vi "Straight Drive.vi"(0 "X":dbl, 1 "Y":dbl, 2 "Z":dbl, 3 "Straight?":bool, 4 "Reverse?":bool) -> (5 "Axes Magnitudes":cluster{"X":dbl, "Y":dbl, "Z":dbl})   [LabVIEW 2016]
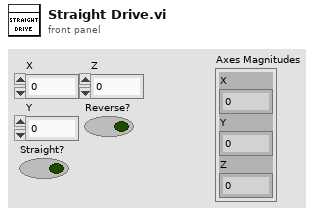
[diagram p1: front panel]
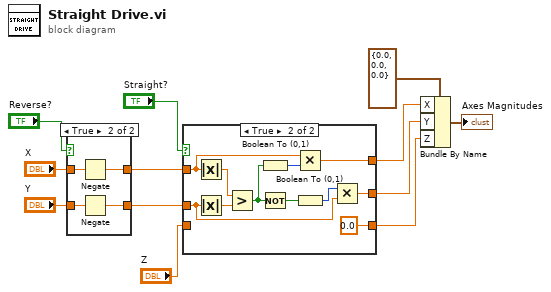
[diagram p0: block diagram]
diagram:
  n1 = case shown="True" "Reverse?" {
    tunnel: [w14 w16] -> w6
    tunnel: "X" -> [w14 w18]
    tunnel: [w13 w17] -> w7
    tunnel: "Y" -> [w13 w15]
    frame False {
    }
    frame True {
      n2 = Negate(x=w18) -> (-x=w16:dbl)
      n3 = Negate(x=w15) -> (-x=w17:dbl)
    }
  }
  n4 = case shown="True" "Straight?" {
    tunnel: w6 -> [w21 w30]
    tunnel: w7 -> [w20 w25]
    tunnel: "Z" -> [w19 _]
    tunnel: [w21 w32] -> w11
    tunnel: [w19 0.0] -> w8
    tunnel: [w20 w31] -> w10
    frame False {
    }
    frame True {
      n5 = Absolute Value(x=w30) -> (abs(x)=w24:dbl)
      n6 = Absolute Value(x=w25) -> (abs(x)=w23:dbl)
      n7 = Greater?(x=w24, y=w23) -> (0:w28:bool)
      n8 = Boolean To (0,1)(Boolean=w28) -> (0, 1=w29:i16)
      n9 = Not(x=w28) -> (.not. x?=w27:bool)
      n10 = Multiply(x=w30, y=w29) -> (x*y=w32:dbl)
      n11 = Boolean To (0,1)(Boolean=w27) -> (0, 1=w26:i16)
      n12 = Multiply(x=w26, y=w25) -> (x*y=w31:dbl)
    }
  }
  n13 = Bundle By Name(cluster=cluster{"X":dbl, "Y":dbl, "Z":dbl} {"X"=0.0, "Y"=0.0, "Z"=0.0} ("input cluster"), "X"=w11, "Y"=w10, "Z"=w8) -> (→"Axes Magnitudes":cluster{"X":dbl, "Y":dbl, "Z":dbl})
